vi "Simple Notifier.vi"() -> ()   [LabVIEW 2023]
doc: "This VI uses a notifier to pass data between parallel loops. Notifiers are most useful when you need to broadcast data from one data source to one or more parallel data sinks."
panel:
  out "Data 2":dbl(graph)
  out "Data 1":dbl(graph)
  in  "Stop":bool
  # "Overview: Demonstrates the use of the Notifier functions to pass data between parallel loops.\nInstructions:\nRun the VI."
  # "The data generated by Loop 1 on the diagram is passed to Loop 2 through a notifier. The stop condition is also monitored in Loop 1 and sent to Loop 2 in a notifier."
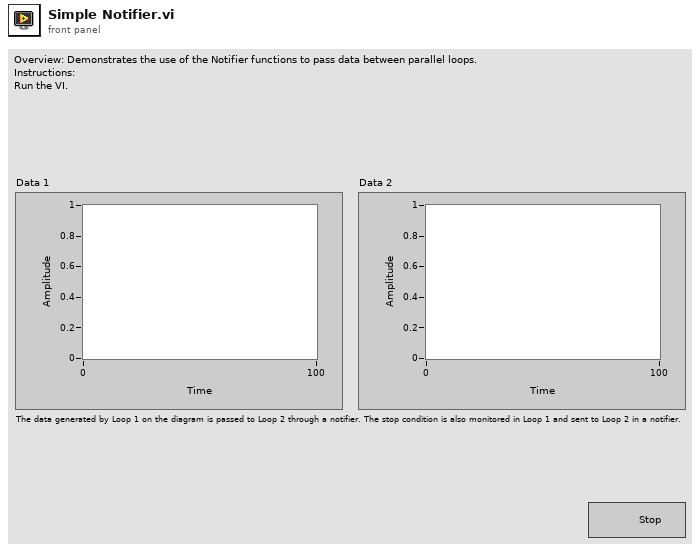
[diagram p1: front panel]
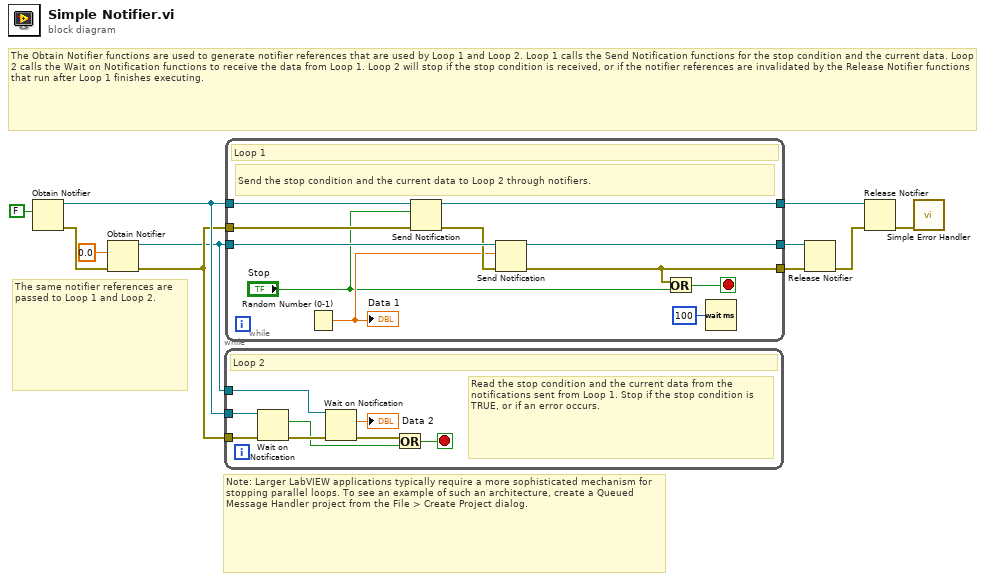
[diagram p0: block diagram]
diagram:
  # "Note: Larger LabVIEW applications typically require a more sophisticated mechanism for stopping parallel loops. To see an example of such an architecture, create a Queued Message Handler project from the File > Create Project dialog."
  # "The same notifier references are passed to Loop 1 and Loop 2."
  # "The Obtain Notifier functions are used to generate notifier references that are used by Loop 1 and Loop 2. Loop 1 calls the Send Notification functions for the stop condition and the current data. Loop 2 calls the Wait on Notification functions to receive the data from Loop 1. Loop 2 will stop if the stop condition is received, or if the notifier references are invalidated by the Release Notifier functions that run after Loop 1 finishes executing."
  n1 = Obtain Notifier(notification data type=FALSE) -> (notifier out=w11:refnum<notifier>, error out=w9:errorcluster)  [unwired: 3 in, 1 out]
  n2 = Obtain Notifier(notification data type=0.0, error in (no error)=w9) -> (notifier out=w1:refnum<notifier>, error out=w2:errorcluster)  [unwired: 2 in, 1 out]
  n3 = while {
    tunnel: w11 -> [w18]
    tunnel: w2 -> [w19]
    tunnel: w1 -> [w16]
    stop <- w12 stop-if-true
    # "Read the stop condition and the current data from the notifications sent from Loop 1. Stop if the stop condition is TRUE, or if an error occurs."
    # "Loop 2"
    n4 = Wait on Notification(notifier=w18, error in (no error)=w19) -> (notification=w13:bool, error out=w17:errorcluster)  [unwired: 2 in, 2 out]
    n5 = Wait on Notification(notifier=w16, error in (no error)=w17) -> (notification=→"Data 2":dbl, error out=w14:errorcluster)  [unwired: 2 in, 2 out]
    n6 = Or(x=w14, y=w13) -> (x .or. y?=w12:bool)
  }
  n7 = while {
    tunnel: w11 -> [w29]
    tunnel: w2 -> [w28]
    tunnel: [w27] -> w4
    tunnel: w1 -> [w26]
    tunnel: [w24] -> w6
    tunnel: [w22] -> w7
    stop <- w20 stop-if-true
    # "Send the stop condition and the current data to Loop 2 through notifiers."
    # "Loop 1"
    n8 = Random Number (0-1)() -> (number: 0 to 1=w23:dbl)
    "Data 1" <- w23
    n9 = Send Notification(notification="Stop", notifier=w29, error in (no error)=w28) -> (notifier out=w27:refnum<notifier>, error out=w25:errorcluster)
    n10 = Send Notification(notification=w23, notifier=w26, error in (no error)=w25) -> (notifier out=w24:refnum<notifier>, error out=w22:errorcluster)
    n11 = Or(x=w22, y="Stop") -> (x .or. y?=w20:bool)
    n12 = Wait (ms)(milliseconds to wait=u32 100) -> ()  [unwired: 1 out]
  }
  n13 = Release Notifier(notifier=w6, error in (no error)=w7) -> (error out=w5:errorcluster)  [unwired: 1 in, 2 out]
  n14 = Release Notifier(notifier=w4, error in (no error)=w5) -> (error out=w3:errorcluster)  [unwired: 1 in, 2 out]
  n15 = call <vilib>:"Simple Error Handler.vi"("error in (no error)"=w3) -> ()  [unwired: 4 in, 5 out]
